vi "MultiBinding.vi"() -> ()   [LabVIEW 2020, in "Examples.lvlib"]
uses:
  Examples.lvlib
  Network Config/Network Config.lvclass
  Server Config/Server Config.lvclass
  PropertyBinder/MultiBinding/MultiBinding.lvclass/MultiBinding.ctl
  PropertyBinder/Binding/Binding.lvclass/Binding.ctl
  PropertyBinder/Transfer Multiple.vi
  PropertyBinder/Binding/Set.vi
  PropertyBinder/Binding/Get.vi
  PropertyBinder/Binding/Binding.lvclass
  PropertyBinder/MultiBinding/MultiBinding.lvclass
panel:
  out "Time":dbl
  out "error out":errorcluster
  out "Bind Port":u16
  out "Bind Address":string
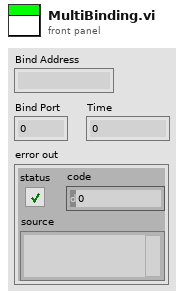
[diagram p1: front panel]
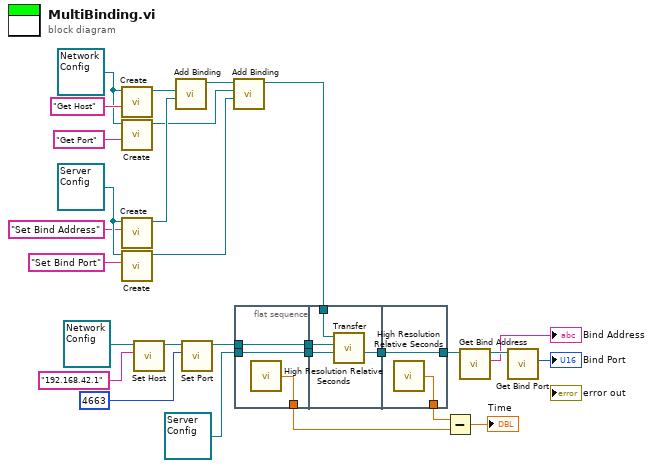
[diagram p0: block diagram]
diagram:
  w23 = refnum<class "Server Config.lvclass"> refnum ("Examples.lvlib:Server Config.lvclass")
  w24 = refnum<class "Network Config.lvclass"> refnum ("Examples.lvlib:Network Config.lvclass")
  n1 = call "Create.vi"("Getter VI Name"="Get Host", "Class Type"=w24) -> ("Binding out"=w8:refnum<class "Binding.lvclass">)  [unwired: 8 in, 1 out]
  n2 = call "Create.vi"("Getter VI Name"="Get Port", "Class Type"=w24) -> ("Binding out"=w5:refnum<class "Binding.lvclass">)  [unwired: 8 in, 1 out]
  n3 = call "Create.vi"("Setter VI Name"="Set Bind Address" ("Getter VI Name"), "Class Type"=w23) -> ("Binding out"=w7:refnum<class "Binding.lvclass">)  [unwired: 8 in, 1 out]
  n4 = call "Create.vi"("Setter VI Name"="Set Bind Port", "Class Type"=w23) -> ("Binding out"=w4:refnum<class "Binding.lvclass">)  [unwired: 8 in, 1 out]
  n5 = call "Set Host.vi"("Host"="192.168.42.1", "Network Config in"=refnum<class "Network Config.lvclass"> refnum ("Examples.lvlib:Network Config.lvclass")) -> ("Network Config out"=w18:refnum<class "Network Config.lvclass">)  [unwired: 8 in, 1 out]
  n6 = call "Add Binding.vi"("Sink"=w7, "Source"=w8) -> ("MultiBinding out"=w6:refnum<class "MultiBinding.lvclass">)  [unwired: 8 in, 1 out]
  n7 = call "Set Port.vi"("Port"=u16 4663, "Network Config in"=w18) -> ("Network Config out"=w13:refnum<class "Network Config.lvclass">)  [unwired: 8 in, 1 out]
  n8 = call "Add Binding.vi"("Sink"=w4, "Source"=w5, "MultiBinding in (New)"=w6) -> ("MultiBinding out"=w1:refnum<class "MultiBinding.lvclass">)  [unwired: 7 in, 1 out]
  n9 = flat-sequence {
    tunnel: refnum<class "Server Config.lvclass"> refnum ("Examples.lvlib:Server Config.lvclass") -> [w30]
    tunnel: w13 -> [w31]
    tunnel: [w31] -> w28
    tunnel: [w30] -> w27
    tunnel: [w29] -> w10
    tunnel: w28 -> [w35]
    tunnel: w27 -> [w34]
    tunnel: [w33] -> w2
    tunnel: w1 -> [w32]
    tunnel: [w37] -> w11
    tunnel: [w36] -> w3
    tunnel: w2 -> [w36]
    frame #0 {
      n10 = call <vilib>:"High Resolution Relative Seconds.vi"() -> ("relative seconds"=w29:dbl)
    }
    frame #1 {
      n11 = call "Transfer.vi"("To Class in"=w34, "From Class in"=w35, "MultiBinding in"=w32) -> ("To Class out"=w33:refnum<class "Server Config.lvclass">)  [unwired: 6 in, 2 out]
    }
    frame #2 {
      n12 = call <vilib>:"High Resolution Relative Seconds.vi"() -> ("relative seconds"=w37:dbl)
    }
  }
  n13 = Subtract(x=w11, y=w10) -> (x-y=→"Time":dbl)
  n14 = call "Get Bind Address.vi"("Server Config in"=w3) -> ("Bind Address"=→"Bind Address":string, "Server Config out"=w16:refnum<class "Server Config.lvclass">)  [unwired: 8 in, 1 out]
  n15 = call "Get Bind Port.vi"("Server Config in"=w16) -> ("Bind Port"=→"Bind Port":u16)  [unwired: 8 in, 2 out]
